vi "Launch Server Loop.vi"(8 "error in (no error)":errorcluster, 11 "Websocket Server in":refnum<class "Websocket Server.lvclass">) -> (0 "error out":errorcluster, 3 "Websocket Server out":refnum<class "Websocket Server.lvclass">)   [LabVIEW 2020, in "Stream-Websocket.lvlib" / "Websocket Server.lvclass"]
uses:
  Websocket Server.lvclass
  Server Loop Async.vi
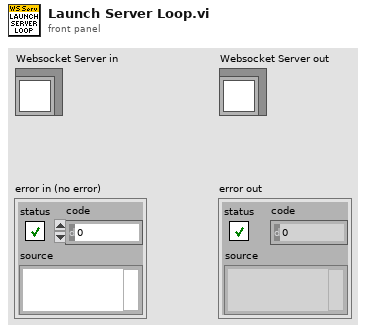
[diagram p1: front panel]
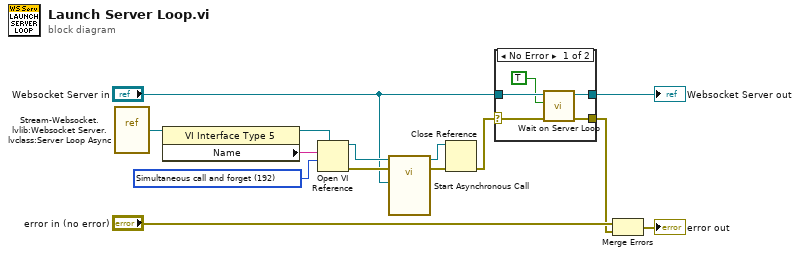
[diagram p0: block diagram]
diagram:
  w8 = 192 items=["Record modifications"=1, "Open templates for editing"=2, "Prompt user to save"=4, "Prepare for reentrant run"=8, "Prompt to find missing subVIs"=16, "Hide loading dialog box"=32, "Enable simultaneous calls"=64, "Prepare to call and forget"=128, "Simultaneous call and forget"=192, "Prepare to call and collect"=256, "Simultaneous call and collect"=320]
  n1 = vi-ref "Stream-Websocket.lvlib:Websocket Server.lvclass:Server Loop Async.vi"() -> (w6:refnum<vi>)
  n2 = property class="VI Interface Type 5"(reference=w6) -> (reference out=w9:refnum<vi>, "Name"=w7:string)  [unwired: 1 in, 1 out]
  n3 = Open VI Reference(type specifier VI Refnum (for type only)=w9, vi path=w7, options=w8) -> (vi reference=w11:refnum<vi>, error out=w10:errorcluster)  [unwired: 3 in]
  n4 = call-by-ref "Start Asynchronous Call"(reference=w11, error in=w10, "Websocket Server in"="Websocket Server in") -> (reference out=w13:refnum<vi>, error out=w12:errorcluster)  [unwired: 11 in]
  n5 = Close Reference(reference=w13, error in (no error)=w12) -> (error out=w4:errorcluster)
  n6 = case shown="No Error" w4 {
    selector: w4 -> [w15 w21]
    tunnel: "Websocket Server in" -> [w19 w20]
    tunnel: [w18 w20] -> w14
    tunnel: [w17 w21] -> w1
    frame No Error {
      n7 = call "Wait on Server Loop.vi"("error in (no error)"=w15, "Value"=TRUE, "Websocket Server in"=w19) -> ("error out"=w17:errorcluster, "Websocket Server out"=w18:refnum<class "Websocket Server.lvclass">)  [unwired: 7 in]
    }
    frame Error {
    }
  }
  "Websocket Server out" <- w14
  n8 = Merge Errors("error in (no error)", w1) -> (→"error out":errorcluster)
